vi "Get Variant Message.vi"(8 "error in (no error)":errorcluster, 11 "Message Double in":refnum<class "Message Double and Boolean Array.lvclass">) -> (0 "error out":errorcluster, 1 "Value":variant, 2 "Name":string, 3 "Message Double out":refnum<class "Message Double and Boolean Array.lvclass">)   [LabVIEW 2016, in "WebSocket Networking.lvlib" / "Message Double and Boolean Array.lvclass"]
doc: "--\nCopyright © 2017 Composed SystemsI All rights reserved.\n\nAuthor: Jon McBee <jon.mcbee@composed.io>\n\nThis library is provided \"AS IS\" ,WITHOUT WARRANTIES OR\nCONDITIONS OF ANY KIND, either express or implied.\n\nComposed Systems -- composed.io\n\nStream 0.0.1.1\nJon McBee - Composed Systems\nCopyright (c) 2017, Composed Systems"
uses:
  <userlib>/Common Components/WebSocket Networking/Message Double and Boolean Array/Message Double and Boolean Array.lvclass
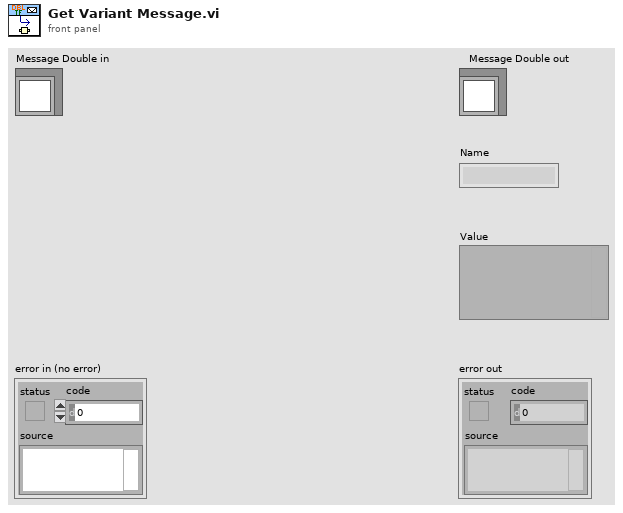
[diagram p1: front panel]
types:
  T1 = typedef "WebSocket Networking.lvlib/Message Double and Boolean Array.lvclass/Value.ctl" = cluster{"Master ID":string, "Doubles":dbl[], "Booleans":bool[]}
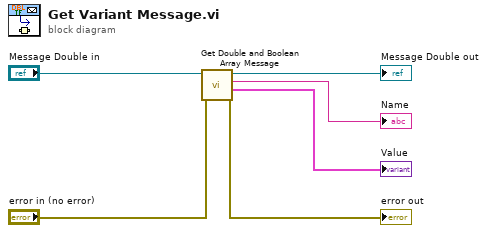
[diagram p0: block diagram]
diagram:
  n1 = call <userlib>:"Get Double and Boolean Array Message.vi"("error in (no error)"="error in (no error)", "Message Double in"="Message Double in") -> ("error out"=→"error out":errorcluster, "Value"=→"Value":T1, "Name"=→"Name":string, "Message Double out"=→"Message Double out":refnum<class "Message Double and Boolean Array.lvclass">)  [unwired: 6 in]
